vi "aided ödev.vi"() -> ()   [LabVIEW 2017]
uses:
  <vilib>/MakerHub/LINX/Public/Peripherals/Analog/Analog Read 1 Chan.vi
  <vilib>/MakerHub/LINX/Public/Peripherals/Analog/Analog Read N Chans.vi
  <vilib>/MakerHub/LINX/Private/Local IO/LinxAnalogRead.vi
  <vilib>/MakerHub/LINX/Public/Utilities/Check Channel.vi
  <vilib>/MakerHub/LINX/Public/Utilities/Open Serial.vi
  <vilib>/MakerHub/LINX/Private/Utilties/Generate Error.vi
  <vilib>/MakerHub/LINX/LMH-LINX.lvlib
panel:
  out "Waveform Chart":dbl(graph)
  out "Thermometer":dbl(slide) scale=0.0..100.0
  in  "Stop":bool
  out "Temperature":dbl
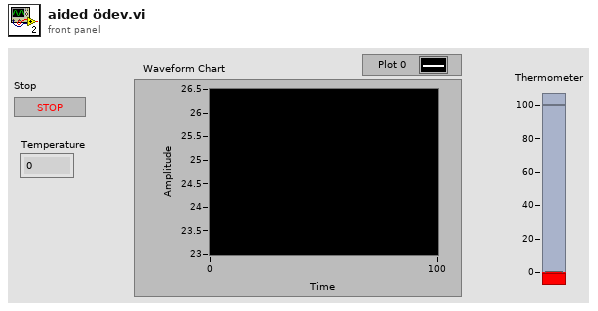
[diagram p1: front panel]
types:
  T1 = typedef "LMH-LINX.lvlib/LINX Ref.ctl" = cluster{"IO":T2, "Interface":T3, "LINX Device Config":T4}
  T2 = typedef "LMH-LINX.lvlib/Platform.ctl" = enum16{"Remote", "Local"}
  T3 = typedef "LMH-LINX.lvlib/Interface.ctl" = enum16{"Serial", "TCP"}
  T4 = typedef "LMH-LINX.lvlib/Device.lvlib/LINX Device Config.ctl" = cluster{"Interface":T3, "COM Port":refnum<visa-resource-name>, "TCP Configuration":T5, "Device Family":u8, "Device ID":u8, "Device Name":string, "TCP Ref":refnum<k5>, "Channels":T6}
  T5 = typedef "LMH-LINX.lvlib/Device.lvlib/TCP Config.ctl" = cluster{"IP Address":string, "Port":u16}
  T6 = typedef "LMH-LINX.lvlib/Channels.ctl" = cluster{"DI":u8[], "DO":u8[], "AI":u8[], "AO":u8[], "PWM":u8[], "QE":u8[], "UART":u8[], "I2C 2":u8[], "SPI":u8[], "CAN":u8[], "Servo":u8[], "AI Ref (V)":dbl, "AI Resolution (Bits)":u8, "AO Ref (V)":dbl, "AO Resolution (Bits)":u8}
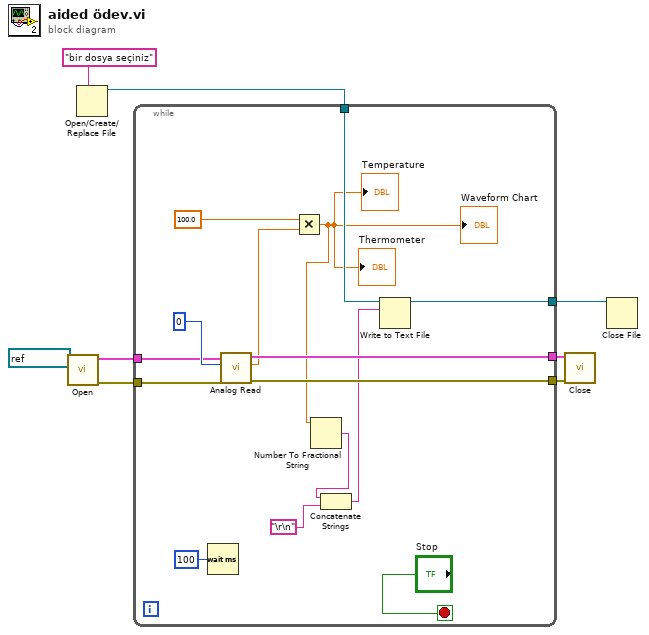
[diagram p0: block diagram]
diagram:
  n1 = call-poly <vilib>:"Open.vi"("Serial Port"=refnum<visa-resource-name> "COM7") -> ("Error Out"=w4:errorcluster, "LINX Resource"=w5:T1)  [unwired: 8 in, 1 out]
  n2 = Open/Create/Replace File(prompt="bir dosya seçiniz") -> (refnum out=w2:refnum<file>)  [unwired: 5 in, 2 out]
  n3 = while {
    tunnel: [w20] -> w8
    tunnel: [w19] -> w7
    tunnel: w5 -> [w18]
    tunnel: w4 -> [w17]
    tunnel: w2 -> [w16]
    tunnel: [w15] -> w1
    stop <- "Stop" stop-if-true
    n4 = Wait (ms)(milliseconds to wait=u32 100) -> ()  [unwired: 1 out]
    n5 = call-poly <vilib>:"Analog Read.vi"("Error In"=w17, "Analog Channel"=u8 0, "LINX Resource"=w18) -> ("Error Out"=w19:errorcluster, "Voltage"=w10:dbl, "LINX Resource"=w20:T1)  [unwired: 5 in, 1 out]
    n6 = Multiply(x=100.0, y=w10) -> (x*y=w9:dbl)
    "Temperature" <- w9
    "Thermometer" <- w9
    "Waveform Chart" <- w9
    n7 = Number To Fractional String(number=w9) -> (F-format string=w12:string)  [unwired: 3 in]
    n8 = Concatenate Strings(w12, "\r\n") -> (w13:string)
    n9 = Write to Text File(file (use dialog)=w16, text=w13) -> (refnum out=w15:refnum<file>)  [unwired: 2 in, 2 out]
  }
  n10 = call <vilib>:"Close.vi"("Error In"=w7, "LINX Resource"=w8) -> ()  [unwired: 9 in, 1 out]
  n11 = Close File(refnum=w1) -> ()  [unwired: 1 in, 2 out]
